vi "networkCheck.vi"() -> (0 "error out":errorcluster, 1 "standard output":string, 2 "standard error":string, 3 "return code":i32)   [LabVIEW 2018]
panel:
  out "T button?":bool
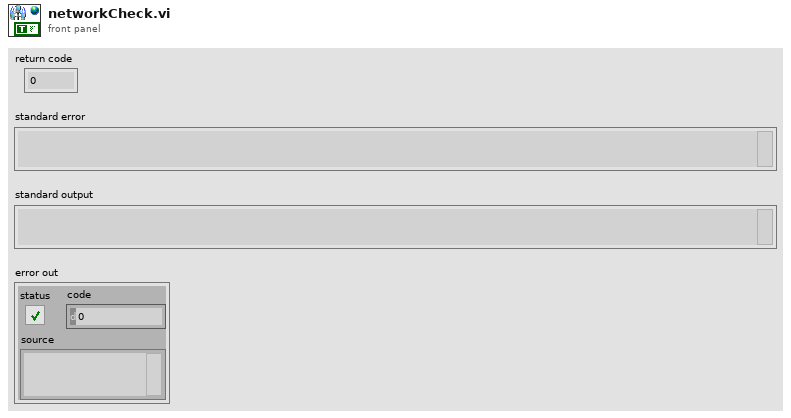
[diagram p1: front panel]
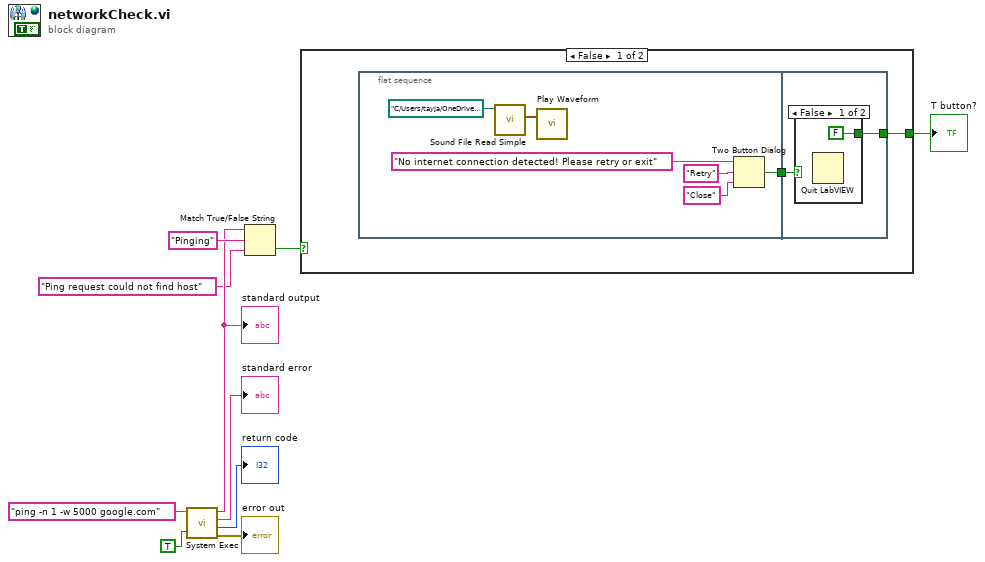
[diagram p0: block diagram]
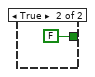
[diagram p2: hidden frame]
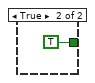
[diagram p3: hidden frame]
diagram:
  n1 = call <vilib>:"System Exec.vi"("run minimized? (F)"=TRUE, "command line"="ping -n 1 -w 5000 google.com") -> ("error out"=→"error out":errorcluster, "return code"=→"return code":i32, "standard error"=→"standard error":string, "standard output"=w8:string)  [unwired: 6 in]
  "standard output" <- w8
  n2 = Match True/False String(2:"Ping request could not find host" ("false string"), 3:"Pinging" ("true string"), 4:w8) -> (0:w10:bool)  [unwired: 1 out]
  n3 = case shown="False" w10 {
    tunnel: [w12 TRUE ("T button?")] -> w1
    frame False {
      n4 = flat-sequence {
        tunnel: [w16] -> w11
        tunnel: [w20] -> w12
        tunnel: w11 -> [w19]
        frame #0 {
          n5 = call <vilib>:"Sound File Read Simple.vi"("path"=path "C:/Users/tayja/OneDrive/Documents/GitHub/adaSuite/lib/media/wav/error.wav") -> ("data"=w17:waveform(dbl)[])  [unwired: 7 in, 3 out]
          n6 = call "Play Waveform"("Data"=w17) -> ()  [unwired: 18 in, 1 out]
          n7 = Two Button Dialog(message="No internet connection detected! Please retry or exit", 1:"Close" ("F button name (\"Cancel\")"), 2:"Retry" ("Left Button Text (\"Yes\")")) -> (T button?=w16:bool)
        }
        frame #1 {
          n8 = case shown="False" w19 {
            tunnel: [FALSE FALSE] -> w20
            frame False {
              n9 = Quit LabVIEW() -> ()  [unwired: 1 in]
            }
            frame True {
            }
          }
        }
      }
    }
    frame True {
    }
  }
  "T button?" <- w1
